vi "Data Execute.vi"(8 "error in (no error)":errorcluster, 10 "Expression":string, 11 "Data DVR in":refnum<data-value>) -> (0 "error out":errorcluster, 2 "Data out":refnum<data-value>, 3 "Data DVR out":refnum<data-value>)   [LabVIEW 2012, in "MDSplus.lvlib"]
doc: "Static method which compiles the expression (via TdiCompile()) and returns the object instance correspondind to the compiled expression."
uses:
  <vilib>/MDSplus/Library/MDSplus.lvlib
  <vilib>/MDSplus/Classes/Data_Class/Data.lvclass
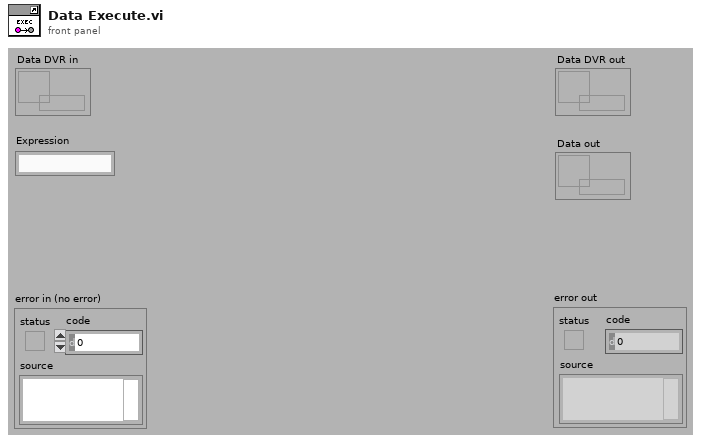
[diagram p1: front panel]
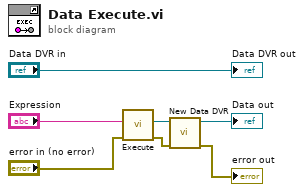
[diagram p0: block diagram]
diagram:
  n1 = call <vilib>:"Execute.vi"("error in (no error)"="error in (no error)", "Expression"="Expression") -> ("error out"=w6:errorcluster, "Returned data out"=w2:refnum<class "Data.lvclass">)  [unwired: 7 in, 1 out]
  n2 = call <vilib>:"New Data DVR.vi"("error in (no error)"=w6, "Data in"=w2) -> ("error out"=→"error out":errorcluster, "Data DVR out"=→"Data out":refnum<data-value>)  [unwired: 8 in]
  "Data DVR out" <- "Data DVR in"
